vi "Go.vi"   [LabVIEW 2014]
uses:
  <vilib>/myRIO/Express VI/Onboard IO/AI/AI Express VI.xnode
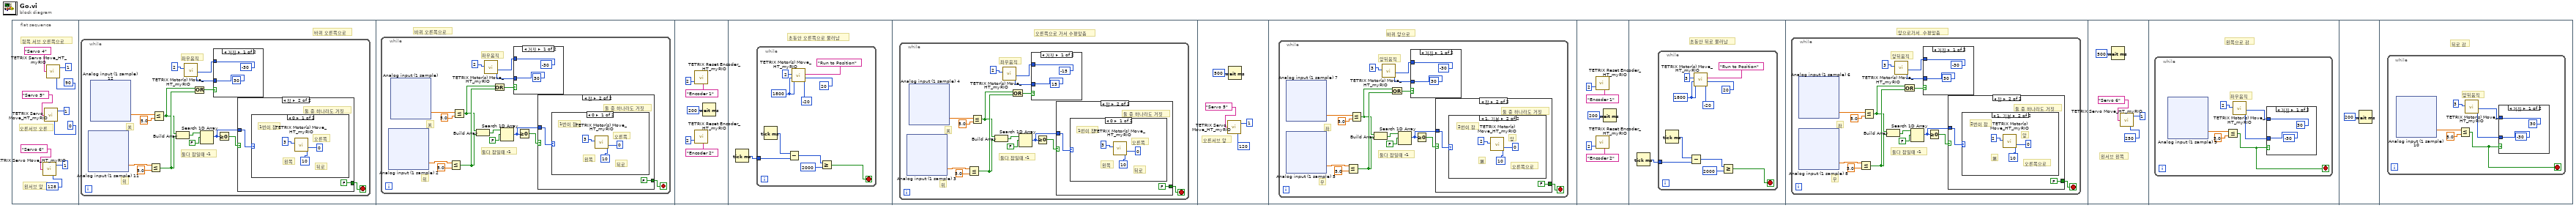
[diagram p0: block diagram]
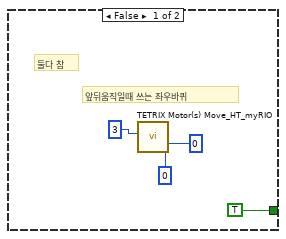
[diagram p2: hidden frame]
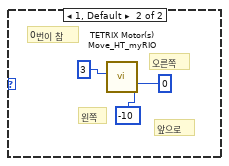
[diagram p3: hidden frame]
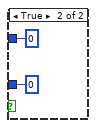
[diagram p4: hidden frame]
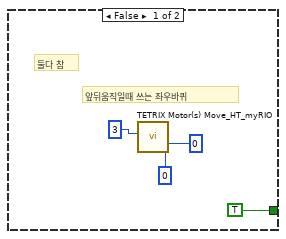
[diagram p5: hidden frame]
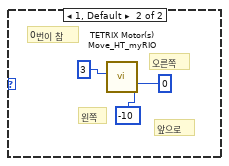
[diagram p6: hidden frame]
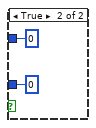
[diagram p7: hidden frame]
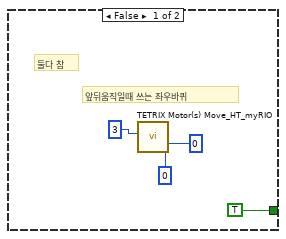
[diagram p8: hidden frame]
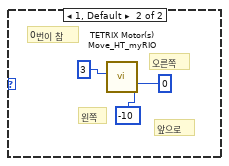
[diagram p9: hidden frame]
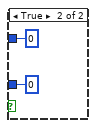
[diagram p10: hidden frame]
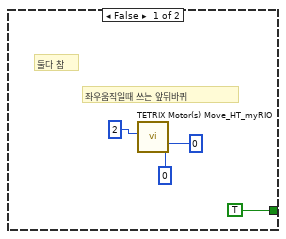
[diagram p11: hidden frame]
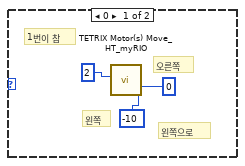
[diagram p12: hidden frame]
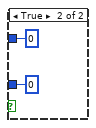
[diagram p13: hidden frame]
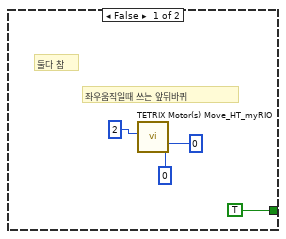
[diagram p14: hidden frame]
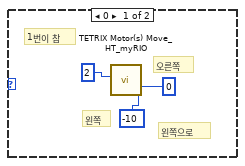
[diagram p15: hidden frame]
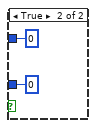
[diagram p16: hidden frame]
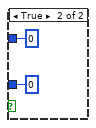
[diagram p17: hidden frame]
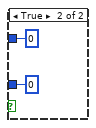
[diagram p18: hidden frame]
diagram:
  n1 = flat-sequence {
    frame #0 {
      # "왼서브 앞"
      # "오른서브 오른"
      # "뒷쪽 서브 오른쪽으로"
      n2 = call <vilib>:"TETRIX Servo Move_HT_myRIO.vi"("Servo Position (0 - 255)"=u8 128, "Controller Daisy Chain Position (1 - 4)"=u8 1, "Select Servo"="Servo 6") -> ()  [unwired: 2 in, 1 out]
      n3 = call <vilib>:"TETRIX Servo Move_HT_myRIO.vi"("Servo Position (0 - 255)"=u8 0, "Controller Daisy Chain Position (1 - 4)"=u8 1, "Select Servo"="Servo 5") -> ()  [unwired: 2 in, 1 out]
      n4 = call <vilib>:"TETRIX Servo Move_HT_myRIO.vi"("Servo Position (0 - 255)"=u8 90, "Controller Daisy Chain Position (1 - 4)"=u8 1, "Select Servo"="Servo 4") -> ()  [unwired: 2 in, 1 out]
    }
    frame #1 {
      # "바퀴 오른쪽으로"
      n5 = while {
        stop <- w10 stop-if-true
        # "关"
        # "위"
        # "둘다 참일때 -1"
        # "좌우움직"
        n6 = xnode "Analog input (1 sample) 11"() -> ("컬러센서1번 (B/AI1 (Pin 5))"=w18:dbl)  [unwired: 1 in, 1 out]
        n7 = xnode "Analog input (1 sample) 12"() -> ("컬러센서0번 (B/AI0 (Pin 3))"=w23:dbl)  [unwired: 1 in, 1 out]
        n8 = Less Or Equal?(x=w18, y=5.0) -> (x <= y?=w12:bool)
        n9 = Less Or Equal?(x=w23, y=5.0) -> (x <= y?=w11:bool)
        n10 = Build Array(w11, w12) -> (w17:bool[])
        n11 = Or(x=w11, y=w12) -> (x .or. y?=w13:bool)
        n12 = Search 1D Array(1D array=w17, element=FALSE ("원소")) -> (index of element=w14:i32)  [unwired: 1 in]
        n13 = case shown="거짓" w13 {
          tunnel: [i8 -30 ("Motor 1 Power (-100 to 100)\n0 = Stop/Brake\n-128 = Stop/Coast") i8 0 ("Motor 1 Power (-100 to 100)\n0 = Stop/Brake\n-128 = Stop/Coast")] -> w21
          tunnel: [i8 30 ("Motor 2 Power (-100 to 100)\n0 = Stop/Brake\n-128 = Stop/Coast") i8 0 ("Motor 2 Power (-100 to 100)\n0 = Stop/Brake\n-128 = Stop/Coast")] -> w20
          frame False {
          }
          frame True {
          }
        }
        n14 = call <vilib>:"TETRIX Motor(s) Move_HT_myRIO.vi"("Motor 2 Power (-100 to 100)\n0 = Stop/Brake\n-128 = Stop/Coast"=w20, "Motor 1 Power (-100 to 100)\n0 = Stop/Brake\n-128 = Stop/Coast"=w21, "Controller Daisy Chain Position: 1 - 4"=u8 2) -> ()  [unwired: 6 in, 1 out]
        n15 = Greater Or Equal To 0?(x=w14) -> (x >= 0?=w15:bool)
        n16 = case shown="참" w15 {
          tunnel: w14 -> [_ w30]
          tunnel: [TRUE FALSE] -> w10
          frame False {
            # "앞뒤움직일때 쓰는 좌우바퀴"
            # "둘다 참"
            n17 = call <vilib>:"TETRIX Motor(s) Move_HT_myRIO.vi"("Motor 2 Power (-100 to 100)\n0 = Stop/Brake\n-128 = Stop/Coast"=i8 0 ("Motor 2 Power (-100 to 100)\n0 = Stop/Brake\n-128 = Stop/Coast"), "Motor 1 Power (-100 to 100)\n0 = Stop/Brake\n-128 = Stop/Coast"=i8 0 ("Motor 1 Power (-100 to 100)\n0 = Stop/Brake\n-128 = Stop/Coast"), "Controller Daisy Chain Position: 1 - 4"=u8 3) -> ()  [unwired: 6 in, 1 out]
          }
          frame True {
            # "둘 중 하나라도 거짓"
            n18 = case shown="0" w30 {
              frame 0 {
                # "뒤로"
                # "왼쪽"
                # "오른쪽"
                # "1번이 참"
                n19 = call <vilib>:"TETRIX Motor(s) Move_HT_myRIO.vi"("Motor 2 Power (-100 to 100)\n0 = Stop/Brake\n-128 = Stop/Coast"=i8 10 ("Motor 2 Power (-100 to 100)\n0 = Stop/Brake\n-128 = Stop/Coast"), "Motor 1 Power (-100 to 100)\n0 = Stop/Brake\n-128 = Stop/Coast"=i8 0 ("Motor 1 Power (-100 to 100)\n0 = Stop/Brake\n-128 = Stop/Coast"), "Controller Daisy Chain Position: 1 - 4"=u8 3) -> ()  [unwired: 6 in, 1 out]
              }
              frame 1, Default {
                # "앞으로"
                # "왼쪽"
                # "오른쪽"
                # "0번이 참"
                n20 = call <vilib>:"TETRIX Motor(s) Move_HT_myRIO.vi"("Motor 2 Power (-100 to 100)\n0 = Stop/Brake\n-128 = Stop/Coast"=i8 -10 ("Motor 2 Power (-100 to 100)\n0 = Stop/Brake\n-128 = Stop/Coast"), "Motor 1 Power (-100 to 100)\n0 = Stop/Brake\n-128 = Stop/Coast"=i8 0 ("Motor 1 Power (-100 to 100)\n0 = Stop/Brake\n-128 = Stop/Coast"), "Controller Daisy Chain Position: 1 - 4"=u8 3) -> ()  [unwired: 6 in, 1 out]
              }
            }
          }
        }
      }
    }
    frame #2 {
      # "바퀴 오른쪽으로"
      n21 = while {
        stop <- w41 stop-if-true
        # "关"
        # "위"
        # "둘다 참일때 -1"
        # "좌우움직"
        n22 = xnode "Analog input (1 sample) 2"() -> ("컬러센서1번 (B/AI1 (Pin 5))"=w49:dbl)  [unwired: 1 in, 1 out]
        n23 = xnode "Analog input (1 sample)"() -> ("컬러센서0번 (B/AI0 (Pin 3))"=w54:dbl)  [unwired: 1 in, 1 out]
        n24 = Less Or Equal?(x=w49, y=5.0) -> (x <= y?=w43:bool)
        n25 = Less Or Equal?(x=w54, y=5.0) -> (x <= y?=w42:bool)
        n26 = Build Array(w42, w43) -> (w48:bool[])
        n27 = Or(x=w42, y=w43) -> (x .or. y?=w44:bool)
        n28 = Search 1D Array(1D array=w48, element=FALSE ("원소")) -> (index of element=w45:i32)  [unwired: 1 in]
        n29 = case shown="거짓" w44 {
          tunnel: [i8 -30 ("Motor 1 Power (-100 to 100)\n0 = Stop/Brake\n-128 = Stop/Coast") i8 0 ("Motor 1 Power (-100 to 100)\n0 = Stop/Brake\n-128 = Stop/Coast")] -> w52
          tunnel: [i8 30 ("Motor 2 Power (-100 to 100)\n0 = Stop/Brake\n-128 = Stop/Coast") i8 0 ("Motor 2 Power (-100 to 100)\n0 = Stop/Brake\n-128 = Stop/Coast")] -> w51
          frame False {
          }
          frame True {
          }
        }
        n30 = call <vilib>:"TETRIX Motor(s) Move_HT_myRIO.vi"("Motor 2 Power (-100 to 100)\n0 = Stop/Brake\n-128 = Stop/Coast"=w51, "Motor 1 Power (-100 to 100)\n0 = Stop/Brake\n-128 = Stop/Coast"=w52, "Controller Daisy Chain Position: 1 - 4"=u8 2) -> ()  [unwired: 6 in, 1 out]
        n31 = Greater Or Equal To 0?(x=w45) -> (x >= 0?=w46:bool)
        n32 = case shown="참" w46 {
          tunnel: w45 -> [_ w61]
          tunnel: [TRUE FALSE] -> w41
          frame False {
            # "앞뒤움직일때 쓰는 좌우바퀴"
            # "둘다 참"
            n33 = call <vilib>:"TETRIX Motor(s) Move_HT_myRIO.vi"("Motor 2 Power (-100 to 100)\n0 = Stop/Brake\n-128 = Stop/Coast"=i8 0 ("Motor 2 Power (-100 to 100)\n0 = Stop/Brake\n-128 = Stop/Coast"), "Motor 1 Power (-100 to 100)\n0 = Stop/Brake\n-128 = Stop/Coast"=i8 0 ("Motor 1 Power (-100 to 100)\n0 = Stop/Brake\n-128 = Stop/Coast"), "Controller Daisy Chain Position: 1 - 4"=u8 3) -> ()  [unwired: 6 in, 1 out]
          }
          frame True {
            # "둘 중 하나라도 거짓"
            n34 = case shown="0" w61 {
              frame 0 {
                # "뒤로"
                # "왼쪽"
                # "오른쪽"
                # "1번이 참"
                n35 = call <vilib>:"TETRIX Motor(s) Move_HT_myRIO.vi"("Motor 2 Power (-100 to 100)\n0 = Stop/Brake\n-128 = Stop/Coast"=i8 10 ("Motor 2 Power (-100 to 100)\n0 = Stop/Brake\n-128 = Stop/Coast"), "Motor 1 Power (-100 to 100)\n0 = Stop/Brake\n-128 = Stop/Coast"=i8 0 ("Motor 1 Power (-100 to 100)\n0 = Stop/Brake\n-128 = Stop/Coast"), "Controller Daisy Chain Position: 1 - 4"=u8 3) -> ()  [unwired: 6 in, 1 out]
              }
              frame 1, Default {
                # "앞으로"
                # "왼쪽"
                # "오른쪽"
                # "0번이 참"
                n36 = call <vilib>:"TETRIX Motor(s) Move_HT_myRIO.vi"("Motor 2 Power (-100 to 100)\n0 = Stop/Brake\n-128 = Stop/Coast"=i8 -10 ("Motor 2 Power (-100 to 100)\n0 = Stop/Brake\n-128 = Stop/Coast"), "Motor 1 Power (-100 to 100)\n0 = Stop/Brake\n-128 = Stop/Coast"=i8 0 ("Motor 1 Power (-100 to 100)\n0 = Stop/Brake\n-128 = Stop/Coast"), "Controller Daisy Chain Position: 1 - 4"=u8 3) -> ()  [unwired: 6 in, 1 out]
              }
            }
          }
        }
      }
    }
    frame #3 {
      n37 = call <vilib>:"TETRIX Reset Encoder_HT_myRIO.vi"("Select Encoder"="Encoder 1", "Controller Daisy Chain Position ( 1 - 4)"=u8 2) -> ()  [unwired: 1 in, 1 out]
      n38 = call <vilib>:"TETRIX Reset Encoder_HT_myRIO.vi"("Select Encoder"="Encoder 2", "Controller Daisy Chain Position ( 1 - 4)"=u8 2) -> ()  [unwired: 1 in, 1 out]
      n39 = Wait (ms)(milliseconds to wait=u32 200 ("대기 시간(ms)")) -> ()  [unwired: 1 out]
    }
    frame #4 {
      # "초동안 오른쪽으로 물러남"
      n40 = Tick Count (ms)() -> (millisecond timer value=w77:u32)
      n41 = while {
        tunnel: w77 -> [w83]
        stop <- w80 stop-if-true
        w85 = 1800 ("Encoder 2 Target: 360 = 1 motor shaft revolution")
        n42 = Tick Count (ms)() -> (millisecond timer value=w84:u32)
        n43 = Subtract(x=w84, y=w83) -> (x-y=w82:u32)
        n44 = call <vilib>:"TETRIX Motor(s) Move_HT_myRIO.vi"("Motor 2 Power (-100 to 100)\n0 = Stop/Brake\n-128 = Stop/Coast"=i8 -20 ("Motor 2 Power (-100 to 100)\n0 = Stop/Brake\n-128 = Stop/Coast"), "Motor 1 Power (-100 to 100)\n0 = Stop/Brake\n-128 = Stop/Coast"=i8 20 ("Motor 1 Power (-100 to 100)\n0 = Stop/Brake\n-128 = Stop/Coast"), "Control Mode"="Run to Position", "Encoder 2 Target: 360 = 1 motor shaft revolution"=w85, "Encoder 1 Target: 360 = 1 motor shaft revolution"=w85, "Controller Daisy Chain Position: 1 - 4"=u8 2) -> ()  [unwired: 3 in, 1 out]
        n45 = Greater Or Equal?(x=w82, y=u32 2000) -> (x >= y?=w80:bool)
      }
    }
    frame #5 {
      # "오른쪽으로 가서 수평맞춤"
      n46 = while {
        stop <- w88 stop-if-true
        # "关"
        # "위"
        # "둘다 참일때 -1"
        # "좌우움직"
        n47 = xnode "Analog input (1 sample) 3"() -> ("컬러센서1번 (B/AI1 (Pin 5))"=w96:dbl)  [unwired: 1 in, 1 out]
        n48 = xnode "Analog input (1 sample) 4"() -> ("컬러센서0번 (B/AI0 (Pin 3))"=w101:dbl)  [unwired: 1 in, 1 out]
        n49 = Less Or Equal?(x=w96, y=5.0) -> (x <= y?=w90:bool)
        n50 = Less Or Equal?(x=w101, y=5.0) -> (x <= y?=w89:bool)
        n51 = Build Array(w89, w90) -> (w95:bool[])
        n52 = Or(x=w89, y=w90) -> (x .or. y?=w91:bool)
        n53 = Search 1D Array(1D array=w95, element=FALSE ("원소")) -> (index of element=w92:i32)  [unwired: 1 in]
        n54 = case shown="거짓" w91 {
          tunnel: [i8 -15 ("Motor 1 Power (-100 to 100)\n0 = Stop/Brake\n-128 = Stop/Coast") i8 0 ("Motor 1 Power (-100 to 100)\n0 = Stop/Brake\n-128 = Stop/Coast")] -> w99
          tunnel: [i8 15 ("Motor 2 Power (-100 to 100)\n0 = Stop/Brake\n-128 = Stop/Coast") i8 0 ("Motor 2 Power (-100 to 100)\n0 = Stop/Brake\n-128 = Stop/Coast")] -> w98
          frame False {
          }
          frame True {
          }
        }
        n55 = call <vilib>:"TETRIX Motor(s) Move_HT_myRIO.vi"("Motor 2 Power (-100 to 100)\n0 = Stop/Brake\n-128 = Stop/Coast"=w98, "Motor 1 Power (-100 to 100)\n0 = Stop/Brake\n-128 = Stop/Coast"=w99, "Controller Daisy Chain Position: 1 - 4"=u8 2) -> ()  [unwired: 6 in, 1 out]
        n56 = Greater Or Equal To 0?(x=w92) -> (x >= 0?=w93:bool)
        n57 = case shown="참" w93 {
          tunnel: w92 -> [_ w108]
          tunnel: [TRUE FALSE] -> w88
          frame False {
            # "앞뒤움직일때 쓰는 좌우바퀴"
            # "둘다 참"
            n58 = call <vilib>:"TETRIX Motor(s) Move_HT_myRIO.vi"("Motor 2 Power (-100 to 100)\n0 = Stop/Brake\n-128 = Stop/Coast"=i8 0 ("Motor 2 Power (-100 to 100)\n0 = Stop/Brake\n-128 = Stop/Coast"), "Motor 1 Power (-100 to 100)\n0 = Stop/Brake\n-128 = Stop/Coast"=i8 0 ("Motor 1 Power (-100 to 100)\n0 = Stop/Brake\n-128 = Stop/Coast"), "Controller Daisy Chain Position: 1 - 4"=u8 3) -> ()  [unwired: 6 in, 1 out]
          }
          frame True {
            # "둘 중 하나라도 거짓"
            n59 = case shown="0" w108 {
              frame 0 {
                # "뒤로"
                # "왼쪽"
                # "오른쪽"
                # "1번이 참"
                n60 = call <vilib>:"TETRIX Motor(s) Move_HT_myRIO.vi"("Motor 2 Power (-100 to 100)\n0 = Stop/Brake\n-128 = Stop/Coast"=i8 10 ("Motor 2 Power (-100 to 100)\n0 = Stop/Brake\n-128 = Stop/Coast"), "Motor 1 Power (-100 to 100)\n0 = Stop/Brake\n-128 = Stop/Coast"=i8 0 ("Motor 1 Power (-100 to 100)\n0 = Stop/Brake\n-128 = Stop/Coast"), "Controller Daisy Chain Position: 1 - 4"=u8 3) -> ()  [unwired: 6 in, 1 out]
              }
              frame 1, Default {
                # "앞으로"
                # "왼쪽"
                # "오른쪽"
                # "0번이 참"
                n61 = call <vilib>:"TETRIX Motor(s) Move_HT_myRIO.vi"("Motor 2 Power (-100 to 100)\n0 = Stop/Brake\n-128 = Stop/Coast"=i8 -10 ("Motor 2 Power (-100 to 100)\n0 = Stop/Brake\n-128 = Stop/Coast"), "Motor 1 Power (-100 to 100)\n0 = Stop/Brake\n-128 = Stop/Coast"=i8 0 ("Motor 1 Power (-100 to 100)\n0 = Stop/Brake\n-128 = Stop/Coast"), "Controller Daisy Chain Position: 1 - 4"=u8 3) -> ()  [unwired: 6 in, 1 out]
              }
            }
          }
        }
      }
    }
    frame #6 {
      # "오른서브 앞"
      n62 = call <vilib>:"TETRIX Servo Move_HT_myRIO.vi"("Servo Position (0 - 255)"=u8 120, "Controller Daisy Chain Position (1 - 4)"=u8 1, "Select Servo"="Servo 5") -> ()  [unwired: 2 in, 1 out]
      n63 = Wait (ms)(milliseconds to wait=u32 500 ("대기 시간(ms)")) -> ()  [unwired: 1 out]
    }
    frame #7 {
      # "바퀴 앞으로"
      n64 = while {
        stop <- w124 stop-if-true
        # "좌"
        # "우"
        # "둘다 참일때 -1"
        # "앞뒤움직"
        n65 = xnode "Analog input (1 sample) 5"() -> ("컬러센서1번 (B/AI1 (Pin 5))"=w132:dbl)  [unwired: 1 in, 1 out]
        n66 = xnode "Analog input (1 sample) 7"() -> ("컬러센서2번 (B/AI2 (Pin 7))"=w123:dbl)  [unwired: 1 in, 1 out]
        n67 = Less Or Equal?(x=w132, y=5.0) -> (x <= y?=w126:bool)
        n68 = Less Or Equal?(x=w123, y=5.0) -> (x <= y?=w125:bool)
        n69 = Build Array(w125, w126) -> (w131:bool[])
        n70 = Or(x=w125, y=w126) -> (x .or. y?=w127:bool)
        n71 = Search 1D Array(1D array=w131, element=FALSE ("원소")) -> (index of element=w128:i32)  [unwired: 1 in]
        n72 = case shown="거짓" w127 {
          tunnel: [i8 -30 ("Motor 1 Power (-100 to 100)\n0 = Stop/Brake\n-128 = Stop/Coast") i8 0 ("Motor 1 Power (-100 to 100)\n0 = Stop/Brake\n-128 = Stop/Coast")] -> w135
          tunnel: [i8 30 ("Motor 2 Power (-100 to 100)\n0 = Stop/Brake\n-128 = Stop/Coast") i8 0 ("Motor 2 Power (-100 to 100)\n0 = Stop/Brake\n-128 = Stop/Coast")] -> w134
          frame False {
          }
          frame True {
          }
        }
        n73 = call <vilib>:"TETRIX Motor(s) Move_HT_myRIO.vi"("Motor 2 Power (-100 to 100)\n0 = Stop/Brake\n-128 = Stop/Coast"=w134, "Motor 1 Power (-100 to 100)\n0 = Stop/Brake\n-128 = Stop/Coast"=w135, "Controller Daisy Chain Position: 1 - 4"=u8 3) -> ()  [unwired: 6 in, 1 out]
        n74 = Greater Or Equal To 0?(x=w128) -> (x >= 0?=w129:bool)
        n75 = case shown="참" w129 {
          tunnel: w128 -> [_ w143]
          tunnel: [TRUE FALSE] -> w124
          frame False {
            # "좌우움직일때 쓰는 앞뒤바퀴"
            # "둘다 참"
            n76 = call <vilib>:"TETRIX Motor(s) Move_HT_myRIO.vi"("Motor 2 Power (-100 to 100)\n0 = Stop/Brake\n-128 = Stop/Coast"=i8 0 ("Motor 2 Power (-100 to 100)\n0 = Stop/Brake\n-128 = Stop/Coast"), "Motor 1 Power (-100 to 100)\n0 = Stop/Brake\n-128 = Stop/Coast"=i8 0 ("Motor 1 Power (-100 to 100)\n0 = Stop/Brake\n-128 = Stop/Coast"), "Controller Daisy Chain Position: 1 - 4"=u8 2) -> ()  [unwired: 6 in, 1 out]
          }
          frame True {
            # "둘 중 하나라도 거짓"
            n77 = case shown="1, 기본" w143 {
              frame 0 {
                # "왼쪽으로"
                # "왼쪽"
                # "오른쪽"
                # "1번이 참"
                n78 = call <vilib>:"TETRIX Motor(s) Move_HT_myRIO.vi"("Motor 2 Power (-100 to 100)\n0 = Stop/Brake\n-128 = Stop/Coast"=i8 -10 ("Motor 2 Power (-100 to 100)\n0 = Stop/Brake\n-128 = Stop/Coast"), "Motor 1 Power (-100 to 100)\n0 = Stop/Brake\n-128 = Stop/Coast"=i8 0 ("Motor 1 Power (-100 to 100)\n0 = Stop/Brake\n-128 = Stop/Coast"), "Controller Daisy Chain Position: 1 - 4"=u8 2) -> ()  [unwired: 6 in, 1 out]
              }
              frame 1, Default {
                # "오른쪽으로"
                # "第"
                # "앞"
                # "2번이 참"
                n79 = call <vilib>:"TETRIX Motor(s) Move_HT_myRIO.vi"("Motor 2 Power (-100 to 100)\n0 = Stop/Brake\n-128 = Stop/Coast"=i8 10 ("Motor 2 Power (-100 to 100)\n0 = Stop/Brake\n-128 = Stop/Coast"), "Motor 1 Power (-100 to 100)\n0 = Stop/Brake\n-128 = Stop/Coast"=i8 0 ("Motor 1 Power (-100 to 100)\n0 = Stop/Brake\n-128 = Stop/Coast"), "Controller Daisy Chain Position: 1 - 4"=u8 2) -> ()  [unwired: 6 in, 1 out]
              }
            }
          }
        }
      }
    }
    frame #8 {
      n80 = call <vilib>:"TETRIX Reset Encoder_HT_myRIO.vi"("Select Encoder"="Encoder 1", "Controller Daisy Chain Position ( 1 - 4)"=u8 2) -> ()  [unwired: 1 in, 1 out]
      n81 = call <vilib>:"TETRIX Reset Encoder_HT_myRIO.vi"("Select Encoder"="Encoder 2", "Controller Daisy Chain Position ( 1 - 4)"=u8 2) -> ()  [unwired: 1 in, 1 out]
      n82 = Wait (ms)(milliseconds to wait=u32 200 ("대기 시간(ms)")) -> ()  [unwired: 1 out]
    }
    frame #9 {
      # "초동안 뒤로 물러남"
      n83 = Tick Count (ms)() -> (millisecond timer value=w159:u32)
      n84 = while {
        tunnel: w159 -> [w165]
        stop <- w162 stop-if-true
        w167 = 1800 ("Encoder 2 Target: 360 = 1 motor shaft revolution")
        n85 = Tick Count (ms)() -> (millisecond timer value=w166:u32)
        n86 = Subtract(x=w166, y=w165) -> (x-y=w164:u32)
        n87 = call <vilib>:"TETRIX Motor(s) Move_HT_myRIO.vi"("Motor 2 Power (-100 to 100)\n0 = Stop/Brake\n-128 = Stop/Coast"=i8 -20 ("Motor 2 Power (-100 to 100)\n0 = Stop/Brake\n-128 = Stop/Coast"), "Motor 1 Power (-100 to 100)\n0 = Stop/Brake\n-128 = Stop/Coast"=i8 20 ("Motor 1 Power (-100 to 100)\n0 = Stop/Brake\n-128 = Stop/Coast"), "Control Mode"="Run to Position", "Encoder 2 Target: 360 = 1 motor shaft revolution"=w167, "Encoder 1 Target: 360 = 1 motor shaft revolution"=w167, "Controller Daisy Chain Position: 1 - 4"=u8 3) -> ()  [unwired: 3 in, 1 out]
        n88 = Greater Or Equal?(x=w164, y=u32 2000) -> (x >= y?=w162:bool)
      }
    }
    frame #10 {
      # "앞으로가서  수평맞춤"
      n89 = while {
        stop <- w171 stop-if-true
        # "좌"
        # "우"
        # "둘다 참일때 -1"
        # "앞뒤움직"
        n90 = xnode "Analog input (1 sample) 8"() -> ("컬러센서1번 (B/AI1 (Pin 5))"=w179:dbl)  [unwired: 1 in, 1 out]
        n91 = xnode "Analog input (1 sample) 6"() -> ("컬러센서2번 (B/AI2 (Pin 7))"=w170:dbl)  [unwired: 1 in, 1 out]
        n92 = Less Or Equal?(x=w179, y=5.0) -> (x <= y?=w173:bool)
        n93 = Less Or Equal?(x=w170, y=5.0) -> (x <= y?=w172:bool)
        n94 = Build Array(w172, w173) -> (w178:bool[])
        n95 = Or(x=w172, y=w173) -> (x .or. y?=w174:bool)
        n96 = Search 1D Array(1D array=w178, element=FALSE ("원소")) -> (index of element=w175:i32)  [unwired: 1 in]
        n97 = case shown="거짓" w174 {
          tunnel: [i8 -30 ("Motor 1 Power (-100 to 100)\n0 = Stop/Brake\n-128 = Stop/Coast") i8 0 ("Motor 1 Power (-100 to 100)\n0 = Stop/Brake\n-128 = Stop/Coast")] -> w182
          tunnel: [i8 30 ("Motor 2 Power (-100 to 100)\n0 = Stop/Brake\n-128 = Stop/Coast") i8 0 ("Motor 2 Power (-100 to 100)\n0 = Stop/Brake\n-128 = Stop/Coast")] -> w181
          frame False {
          }
          frame True {
          }
        }
        n98 = call <vilib>:"TETRIX Motor(s) Move_HT_myRIO.vi"("Motor 2 Power (-100 to 100)\n0 = Stop/Brake\n-128 = Stop/Coast"=w181, "Motor 1 Power (-100 to 100)\n0 = Stop/Brake\n-128 = Stop/Coast"=w182, "Controller Daisy Chain Position: 1 - 4"=u8 3) -> ()  [unwired: 6 in, 1 out]
        n99 = Greater Or Equal To 0?(x=w175) -> (x >= 0?=w176:bool)
        n100 = case shown="참" w176 {
          tunnel: w175 -> [_ w190]
          tunnel: [TRUE FALSE] -> w171
          frame False {
            # "좌우움직일때 쓰는 앞뒤바퀴"
            # "둘다 참"
            n101 = call <vilib>:"TETRIX Motor(s) Move_HT_myRIO.vi"("Motor 2 Power (-100 to 100)\n0 = Stop/Brake\n-128 = Stop/Coast"=i8 0 ("Motor 2 Power (-100 to 100)\n0 = Stop/Brake\n-128 = Stop/Coast"), "Motor 1 Power (-100 to 100)\n0 = Stop/Brake\n-128 = Stop/Coast"=i8 0 ("Motor 1 Power (-100 to 100)\n0 = Stop/Brake\n-128 = Stop/Coast"), "Controller Daisy Chain Position: 1 - 4"=u8 2) -> ()  [unwired: 6 in, 1 out]
          }
          frame True {
            # "둘 중 하나라도 거짓"
            n102 = case shown="1, 기본" w190 {
              frame 0 {
                # "왼쪽으로"
                # "왼쪽"
                # "오른쪽"
                # "1번이 참"
                n103 = call <vilib>:"TETRIX Motor(s) Move_HT_myRIO.vi"("Motor 2 Power (-100 to 100)\n0 = Stop/Brake\n-128 = Stop/Coast"=i8 -10 ("Motor 2 Power (-100 to 100)\n0 = Stop/Brake\n-128 = Stop/Coast"), "Motor 1 Power (-100 to 100)\n0 = Stop/Brake\n-128 = Stop/Coast"=i8 0 ("Motor 1 Power (-100 to 100)\n0 = Stop/Brake\n-128 = Stop/Coast"), "Controller Daisy Chain Position: 1 - 4"=u8 2) -> ()  [unwired: 6 in, 1 out]
              }
              frame 1, Default {
                # "오른쪽으로"
                # "第"
                # "앞"
                # "2번이 참"
                n104 = call <vilib>:"TETRIX Motor(s) Move_HT_myRIO.vi"("Motor 2 Power (-100 to 100)\n0 = Stop/Brake\n-128 = Stop/Coast"=i8 10 ("Motor 2 Power (-100 to 100)\n0 = Stop/Brake\n-128 = Stop/Coast"), "Motor 1 Power (-100 to 100)\n0 = Stop/Brake\n-128 = Stop/Coast"=i8 0 ("Motor 1 Power (-100 to 100)\n0 = Stop/Brake\n-128 = Stop/Coast"), "Controller Daisy Chain Position: 1 - 4"=u8 2) -> ()  [unwired: 6 in, 1 out]
              }
            }
          }
        }
      }
    }
    frame #11 {
      # "왼서브 왼쪽"
      n105 = Wait (ms)(milliseconds to wait=u32 500 ("대기 시간(ms)")) -> ()  [unwired: 1 out]
      n106 = call <vilib>:"TETRIX Servo Move_HT_myRIO.vi"("Servo Position (0 - 255)"=u8 250, "Controller Daisy Chain Position (1 - 4)"=u8 1, "Select Servo"="Servo 6") -> ()  [unwired: 2 in, 1 out]
    }
    frame #12 {
      # "왼쪽으로 감"
      n107 = while {
        stop <- w205 stop-if-true
        # "좌우움직"
        n108 = xnode "Analog input (1 sample) 9"() -> ("컬러센서2번 (B/AI2 (Pin 7))"=w206:dbl)  [unwired: 1 in, 1 out]
        n109 = Less Or Equal?(x=w206, y=5.0) -> (x <= y?=w205:bool)
        n110 = case shown="거짓" w205 {
          tunnel: [i8 30 ("Motor 1 Power (-100 to 100)\n0 = Stop/Brake\n-128 = Stop/Coast") i8 0 ("Motor 1 Power (-100 to 100)\n0 = Stop/Brake\n-128 = Stop/Coast")] -> w208
          tunnel: [i8 -30 ("Motor 2 Power (-100 to 100)\n0 = Stop/Brake\n-128 = Stop/Coast") i8 0 ("Motor 2 Power (-100 to 100)\n0 = Stop/Brake\n-128 = Stop/Coast")] -> w207
          frame False {
          }
          frame True {
          }
        }
        n111 = call <vilib>:"TETRIX Motor(s) Move_HT_myRIO.vi"("Motor 2 Power (-100 to 100)\n0 = Stop/Brake\n-128 = Stop/Coast"=w207, "Motor 1 Power (-100 to 100)\n0 = Stop/Brake\n-128 = Stop/Coast"=w208, "Controller Daisy Chain Position: 1 - 4"=u8 2) -> ()  [unwired: 6 in, 1 out]
      }
    }
    frame #13 {
      n112 = Wait (ms)(milliseconds to wait=u32 200 ("대기 시간(ms)")) -> ()  [unwired: 1 out]
    }
    frame #14 {
      # "뒤로 감"
      n113 = while {
        stop <- w217 stop-if-true
        # "앞뒤움직"
        n114 = xnode "Analog input (1 sample) 10"() -> ("컬러센서1번 (B/AI1 (Pin 5))"=w216:dbl)  [unwired: 1 in, 1 out]
        n115 = Less Or Equal?(x=w216, y=5.0) -> (x <= y?=w217:bool)
        n116 = case shown="거짓" w217 {
          tunnel: [i8 30 ("Motor 1 Power (-100 to 100)\n0 = Stop/Brake\n-128 = Stop/Coast") i8 0 ("Motor 1 Power (-100 to 100)\n0 = Stop/Brake\n-128 = Stop/Coast")] -> w219
          tunnel: [i8 -30 ("Motor 2 Power (-100 to 100)\n0 = Stop/Brake\n-128 = Stop/Coast") i8 0 ("Motor 2 Power (-100 to 100)\n0 = Stop/Brake\n-128 = Stop/Coast")] -> w218
          frame False {
          }
          frame True {
          }
        }
        n117 = call <vilib>:"TETRIX Motor(s) Move_HT_myRIO.vi"("Motor 2 Power (-100 to 100)\n0 = Stop/Brake\n-128 = Stop/Coast"=w218, "Motor 1 Power (-100 to 100)\n0 = Stop/Brake\n-128 = Stop/Coast"=w219, "Controller Daisy Chain Position: 1 - 4"=u8 3) -> ()  [unwired: 6 in, 1 out]
      }
    }
  }
